vi "Process Primary Input.vi"(11 "Ship in":refnum<class "Ship.lvclass">) -> (2 "New Elements":refnum<class "Element.lvclass">[](array[class]), 3 "Ship out":refnum<class "Ship.lvclass">)   [LabVIEW 2021, in "Ship.lvclass"]
uses:
  Ship.lvclass
  Element/Element.lvclass
  Ship.lvclass/Ship.ctl
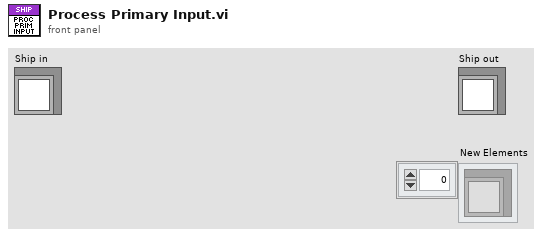
[diagram p1: front panel]
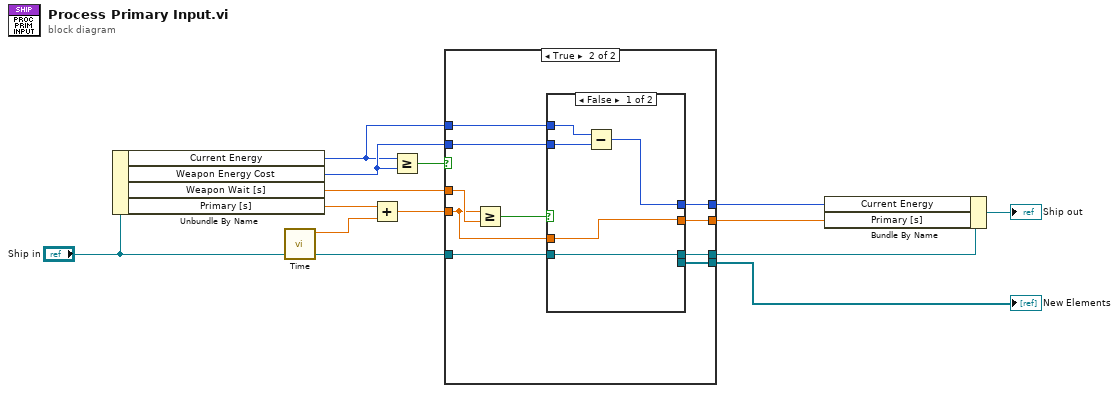
[diagram p0: block diagram]
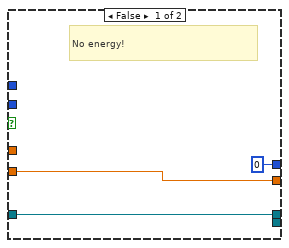
[diagram p2: hidden frame]
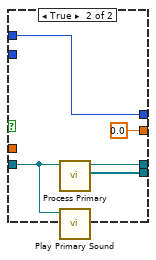
[diagram p3: hidden frame]
diagram:
  n1 = Unbundle By Name("Ship in") -> ("Current Energy"=w3:i32, "Weapon Energy Cost"=w4:i32, "Weapon Wait [s]"=w10:sgl, "Primary [s]"=w11:sgl)
  n2 = call "Time.vi"() -> ("Delta Time [s]"=w12:sgl)  [unwired: 10 in, 1 out]
  n3 = Add(x=w11, y=w12) -> (x+y=w6:sgl)
  n4 = Greater Or Equal?(x=w3, y=w4) -> (x >= y?=w1:bool)
  n5 = case shown="True" w1 {
    tunnel: [_ w26] -> w13
    tunnel: w10 -> [_ w25]
    tunnel: [w14 w24] -> w9
    tunnel: [w16 w23] -> w7
    tunnel: w6 -> [w14 w22]
    tunnel: "Ship in" -> [w16 w21]
    tunnel: w4 -> [_ w20]
    tunnel: w3 -> [_ w19]
    tunnel: [0 ("Current Energy") w18] -> w2
    frame False {
      # "No energy!"
    }
    frame True {
      n6 = Greater Or Equal?(x=w22, y=w25) -> (x >= y?=w17:bool)
      n7 = case shown="False" w17 {
        tunnel: [w30 w36] -> w23
        tunnel: [_ w35] -> w26
        tunnel: w21 -> [w30 w34]
        tunnel: [w31 sgl 0.0] -> w24
        tunnel: w22 -> [w31 _]
        tunnel: w20 -> [w28 _]
        tunnel: w19 -> [w29 w32]
        tunnel: [w27 w32] -> w18
        frame False {
          n8 = Subtract(x=w29, y=w28) -> (x-y=w27:i32)
        }
        frame True {
          n9 = call-dynamic "Process Primary.vi"("Ship in"=w34) -> ("New Elements"=w35:refnum<class "Element.lvclass">[], "Ship out"=w36:refnum<class "Ship.lvclass">)  [unwired: 9 in]
          n10 = call-dynamic "Play Primary Sound.vi"("Ship in"=w34) -> ()  [unwired: 10 in, 1 out]
        }
      }
    }
  }
  "New Elements" <- w13
  n11 = Bundle By Name(cluster=w7, "Current Energy"=w2, "Primary [s]"=w9) -> (→"Ship out":refnum<class "Ship.lvclass">)
